vi "V_F_CorrezioneV.vi"(7 "Limita":bool, 8 "%":dbl=11.5 format="%#_13g", 9 "Fginocchio":dbl, 10 "Vmax":dbl, 11 "Value in":cluster{"Hz":dbl, "V":dbl}) -> (0 "Hz dec":dbl, 1 "Hz int":dbl, 2 "correzione V %":dbl, 3 "Value out":cluster{"Hz":dbl, "V":dbl}, 4 "rif":u16, 6 "In Range?":bool)   [LabVIEW 2019]
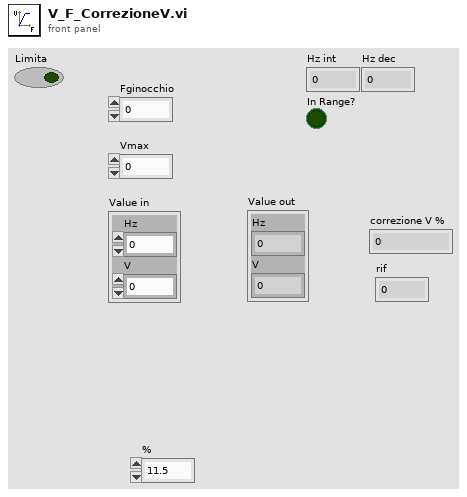
[diagram p1: front panel]
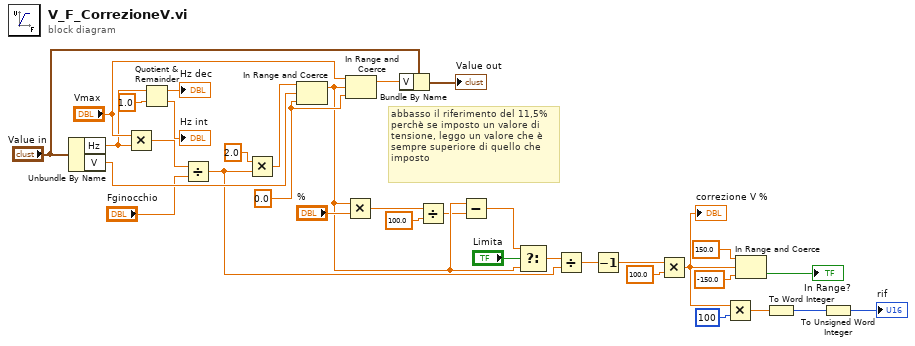
[diagram p0: block diagram]
diagram:
  w29 = 0.0 ("lower limit")
  # "abbasso il riferimento del 11,5%\nperchè se imposto un valore di \ntensione, leggo un valore che è\nsempre superiore di quello che\nimposto"
  n1 = Unbundle By Name("Value in") -> ("Hz"=w21:dbl, "V"=w32:dbl)
  n2 = Multiply(x="Vmax", y=w21) -> (x*y=w30:dbl)
  n3 = Quotient & Remainder(x=w21, y=1.0) -> (x-y*floor(x/y)=→"Hz dec":dbl, floor(x/y)=→"Hz int":dbl)
  n4 = Divide(x=w30, y="Fginocchio") -> (x/y=w12:dbl)
  n5 = Multiply(x=2.0, y=w12) -> (x*y=w25:dbl)
  n6 = In Range and Coerce(upper limit=w25, x=w32, lower limit=w29) -> (coerced(x)=w8:dbl)  [unwired: 1 out]
  n7 = Multiply(x=w8, y="%") -> (x*y=w15:dbl)
  n8 = In Range and Coerce(upper limit="Vmax", x=w8, lower limit=w29) -> (coerced(x)=w27:dbl)  [unwired: 1 out]
  n9 = Bundle By Name(cluster="Value in", "V"=w27) -> (→"Value out":cluster{"Hz":dbl, "V":dbl})
  n10 = Divide(x=w15, y=100.0) -> (x/y=w7:dbl)
  n11 = Subtract(x=w8, y=w7) -> (x-y=w9:dbl)
  n12 = Select(t=w9, s="Limita", f=w8) -> (s? t:f=w10:dbl)
  n13 = Divide(x=w10, y=w12) -> (x/y=w24:dbl)
  n14 = Decrement(x=w24) -> (x-1=w23:dbl)
  n15 = Multiply(x=w23, y=100.0) -> (x*y=w4:dbl)
  "correzione V %" <- w4
  n16 = Multiply(x=w4, y=i16 100) -> (x*y=w13:dbl)
  n17 = In Range and Coerce(upper limit=150.0 ("lower limit"), x=w4, lower limit=-150.0) -> (In Range?=→"In Range?":bool)  [unwired: 1 out]
  n18 = To Word Integer(number=w13) -> (16bit integer=w6:i16)
  n19 = To Unsigned Word Integer(number=w6) -> (unsigned 16bit integer=→"rif":u16)
